vi "UV-VIS SetNumberKinetics.vi"(3 "error in (no error)":errorcluster, 4 "number":i32, 5 "Detector in":refnum<class "CCD_camera.lvclass">) -> (0 "error out":errorcluster, 1 "DLL error code":u32, 2 "Detector out":refnum<class "CCD_camera.lvclass">)   [LabVIEW 2020, in "CCD_camera.lvclass"]
doc: "This function will set the number of scans (possibly accumulated scans) to be taken during a single acquisition sequence. This will only take effect if the acquisition mode is Kinetic Series.\n\n<B>Parameter:</B>\nnumber - number of scans to store\n\n<B>Error codes:</B>\nDRV_SUCCESS - Series length set.\nDRV_NOT_INITIALIZED - System not initialized.\nDRV_ACQUIRING - Acquisition in progress.\nDRV_P1INVALID - Number in series invalid."
uses:
  CCD_camera.lvclass
  C:/dev/TRANCON/Classes/Detector/Detector.lvclass
  Detector.lvclass/Detector.ctl
  Detector.lvclass
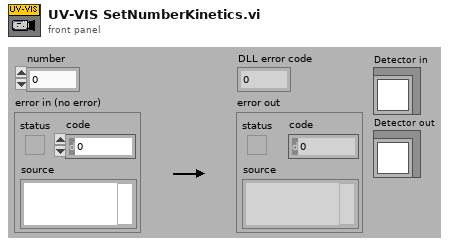
[diagram p1: front panel]
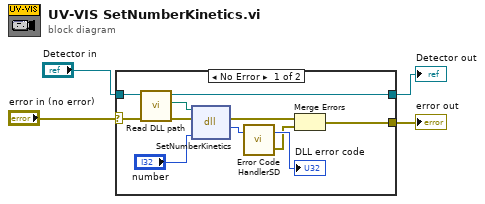
[diagram p0: block diagram]
diagram:
  n1 = case shown="No Error" "error in (no error)" {
    selector: "error in (no error)" -> [w10 w17]
    tunnel: [w6 w17] -> w3
    tunnel: "Detector in" -> [w7 w16]
    tunnel: [w5 w16] -> w1
    frame No Error {
      n2 = call "Read DLL path.vi"("error in (no error)"=w10, "Detector in"=w7) -> ("error out"=w9:errorcluster, "DLL path"=w8:path, "Detector out"=w5:refnum<class "CCD_camera.lvclass">)  [unwired: 7 in]
      n3 = dll-call lib="S:/TRANCON/DLL/Atmcd32d.dll" fn="SetNumberKinetics"(path in=w8, error in=w9, "number"="number") -> (error out=w11:errorcluster, "return type"=w15:u32)  [unwired: 2 in, 1 out]
      n4 = call "Error Code HandlerSD.vi"("DLL error code"=w15) -> ("error out"=w12:errorcluster, "dup DLL error code"=→"DLL error code":u32)  [unwired: 1 in]
      n5 = Merge Errors(w11, w12) -> (w6:errorcluster)
    }
    frame Error {
    }
  }
  "error out" <- w3
  "Detector out" <- w1
